vi "TeachAndPlay_old.vi"() -> ()   [LabVIEW 2013]
uses:
  ROS/Code/JointPositions.ctl
  ROS/Code/SubVIs/BaxterSide.ctl
  ROS/Code/SubVIs/BaxterButtons.ctl
panel:
  in  "Functions":i32[](listbox)=[0, 2, 4]
  out "Gripper State":bool=TRUE
  in  "Path":T2(array[cluster])=[{"Position"={"e0"=0.043945312449785154, "e1"=0.417480468272959, "s0"=0.08789062489957031, "s1"=0.8569335927708106, "w0"=0.08789062489957031, "w1"=0.1318359373493555, "w2"=-0.1098632811244629}, "Name"="Zero", "Gripper"=TRUE}, {"Position"={"e0"=1.6918945293167287, "e1"=3.4497070273081354, "s0"=-1.8017578104411913, "s1"=-4.85595702570126, "w0"=0.06591796867467775, "w1"=87.01171865057462, "w2"=0.2416992184738184}, "Name"="Point Down", "Gripper"=TRUE}, {"Position"={"e0"=3.0, "e1"=26.0, "s0"=-51.0, "s1"=-15.0, "w0"=-4.0, "w1"=77.0, "w2"=-4.0}, "Name"="", "Gripper"=FALSE}, {"Position"={"e0"=3.229980465059209, "e1"=26.257324188746633, "s0"=-51.39404291002375, "s1"=-14.63378904577846, "w0"=-3.7573242144566312, "w1"=76.61865225620042, "w2"=-3.6254882771072756}, "Name"="Approach", "Gripper"=TRUE}, {"Position"={"e0"=4.965820306825724, "e1"=34.760742147780064, "s0"=-53.085937439340476, "s1"=-15.754394513247982, "w0"=-3.999023432930449, "w1"=65.06103508190692, "w2"=-3.889160151805987}, "Name"="Grip", "Gripper"=TRUE}, {"Position"={"e0"=4.987792963050616, "e1"=34.89257808512942, "s0"=-53.21777337668983, "s1"=-15.644531232123517, "w0"=-4.08691405783002, "w1"=65.21484367548118, "w2"=-3.823242183131309}, "Name"="Close", "Gripper"=FALSE}, {"Position"={"e0"=7.031249991965626, "e1"=34.9584960538041, "s0"=-53.085937439340476, "s1"=-26.696777313244485, "w0"=-3.889160151805987, "w1"=74.6191405397352, "w2"=-3.8012695269064167}, "Name"="Withdraw", "Gripper"=FALSE}, {"Position"={"e0"=9.03076170843085, "e1"=46.01074213492506, "s0"=-1.2524414048188772, "s1"=-34.69482417910538, "w0"=-12.76611326666259, "w1"=74.59716788351031, "w2"=9.140624989555315}, "Name"="Swing Away", "Gripper"=FALSE}, {"Position"={"e0"=8.898925771081496, "e1"=45.79101557267614, "s0"=-1.2524414048188772, "s1"=-34.541015585531134, "w0"=-12.875976547787051, "w1"=74.75097647708456, "w2"=9.008789052205957}, "Name"="Drop", "Gripper"=TRUE}] {"Position"."w2" scale=-175.25..175.25; "Position"."w1" scale=-90.0..120.0; "Position"."w0" scale=-175.25..175.25; "Position"."e1" scale=-3.0..150.0; "Position"."e0" scale=-173.5..173.5; "Position"."s1" scale=-123.0..60.0; "Position"."s0" scale=-141.0..51.0}
  in  "Tab":enum32{"Teach", "Edit", "Play", "Save", "Load"}(tab)=enum."Play"
  in  "New Path?":bool
  out "Last Activity":string="---------"
  in  "Pause":bool=TRUE
  in  "Tolerance":dbl=1.0
  in  "Settle Time":u32=2500
  in  "save path":path=path "C:/Program Files/Labview/user.lib/ROSforLV_0.1/Devices/Baxter/Baxter Examples/Paths/Pick.csv"
  in  "Save":bool
  in  "load file":path
  in  "Load":bool
  in  "stop":bool
  # "Not yet"
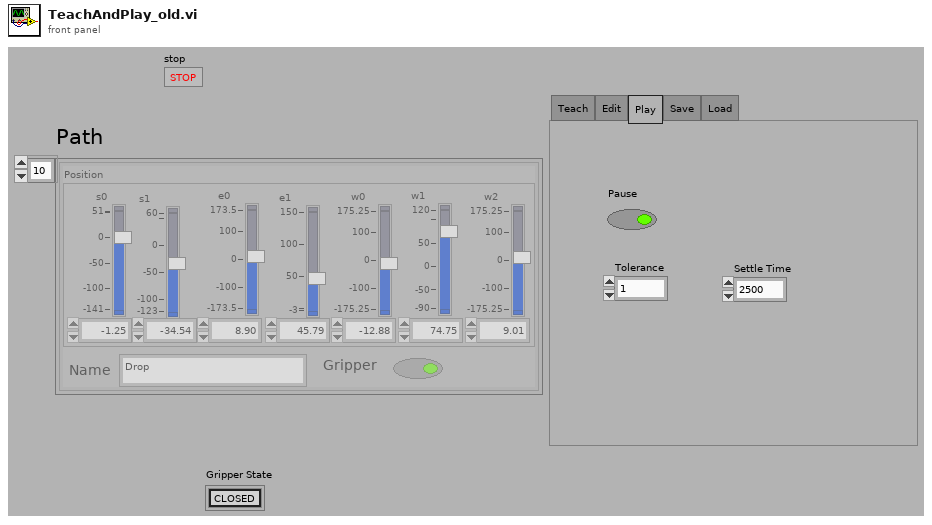
[diagram p1: front panel]
types:
  T1 = typedef "JointPositions.ctl" = cluster{"e0":dbl, "e1":dbl, "s0":dbl, "s1":dbl, "w0":dbl, "w1":dbl, "w2":dbl}
  T2 = cluster{"Position":T1, "Name":string, "Gripper":bool}[]
  T3 = cluster{"Positions":T1, "Name":string, "Gripper":bool}
  T4 = typedef "BaxterSide.ctl" = enum16{"left", "right"}
  T5 = enum16{"open", "replace", "create", "open or create", "replace or create", "replace or create with confirmation"}
  T6 = typedef "BaxterButtons.ctl" = u16
  T7 = cluster{"Cancel":bool, "OK":bool, "Show":bool, "Wheel":u8}
  T8 = cluster{"Positions":T1, "Name":string, "Gripper":bool}[]
  T9 = cluster{"Position":T1, "Name":string, "Gripper":bool}
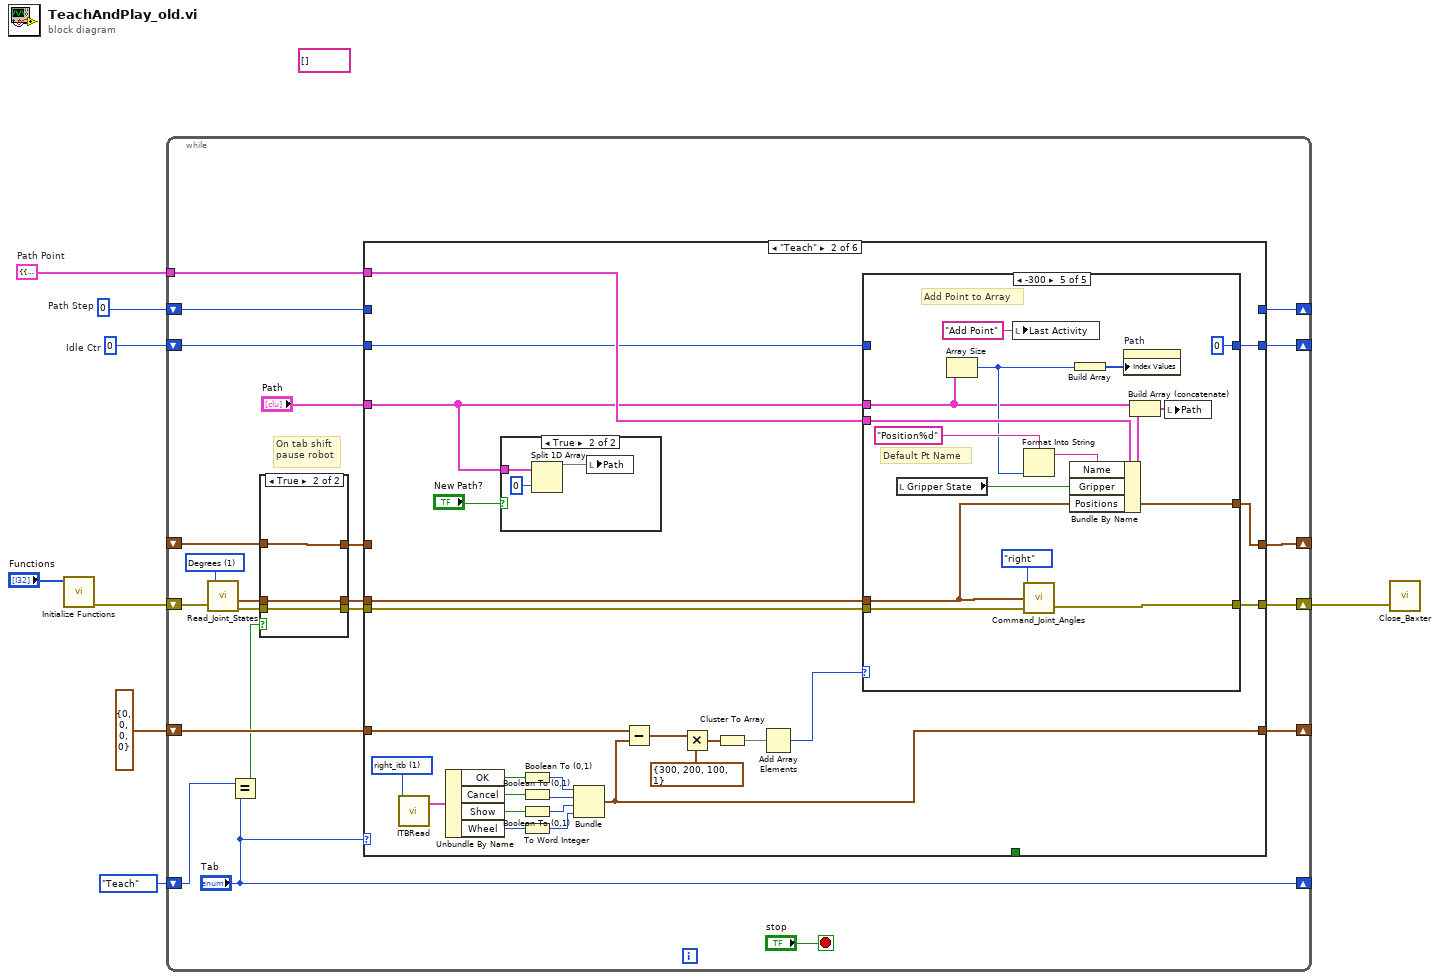
[diagram p0: block diagram]
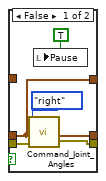
[diagram p2: hidden frame]
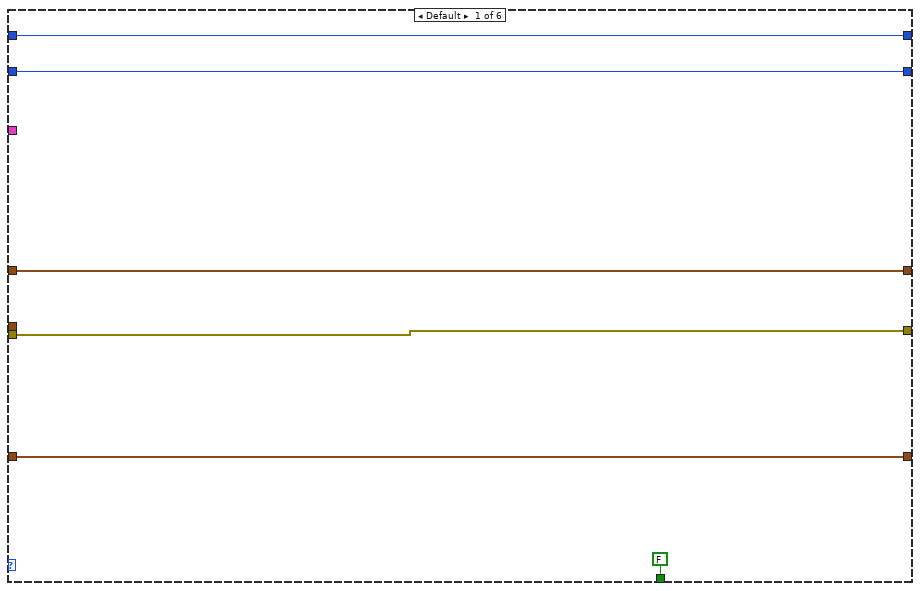
[diagram p3: hidden frame]
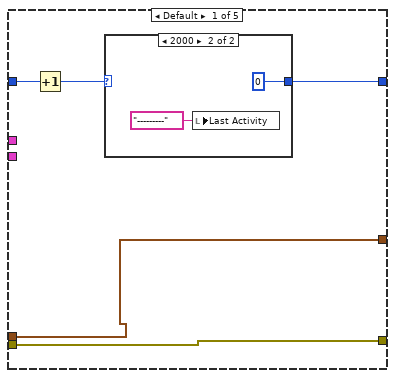
[diagram p5: hidden frame]
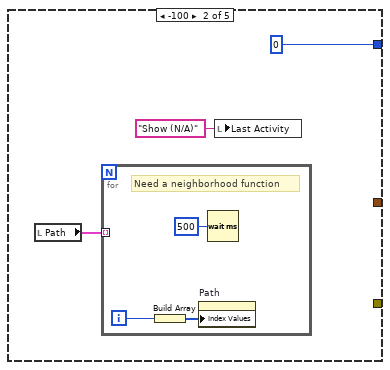
[diagram p7: hidden frame]
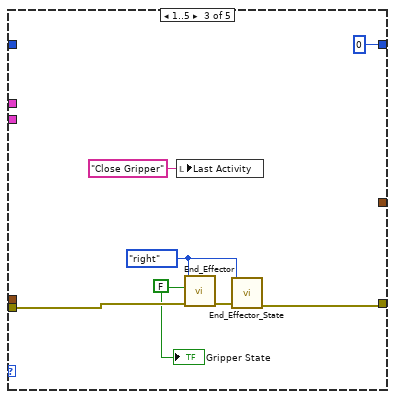
[diagram p8: hidden frame]
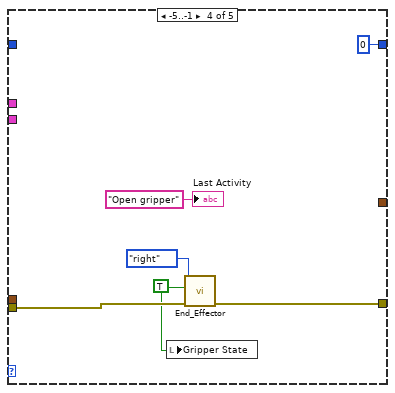
[diagram p9: hidden frame]
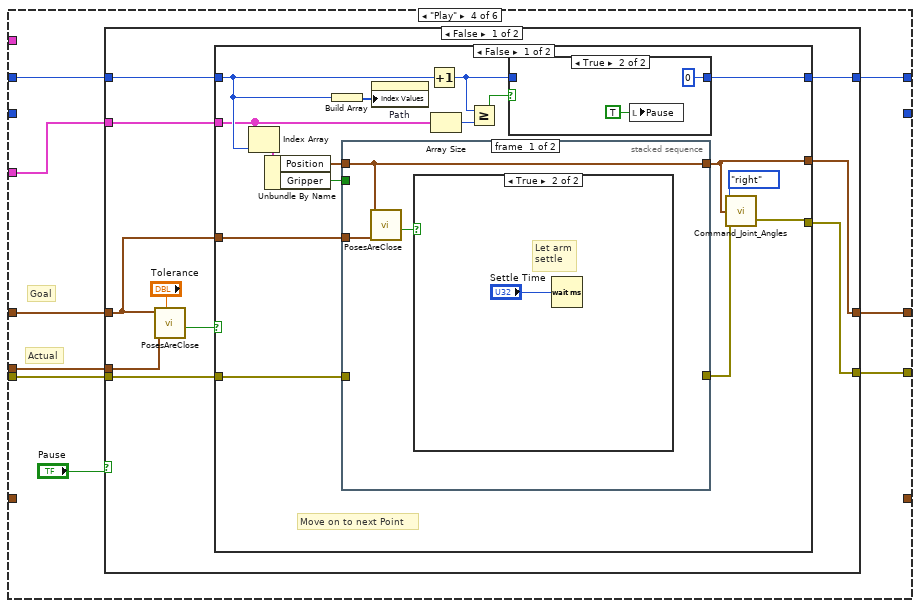
[diagram p11: hidden frame]
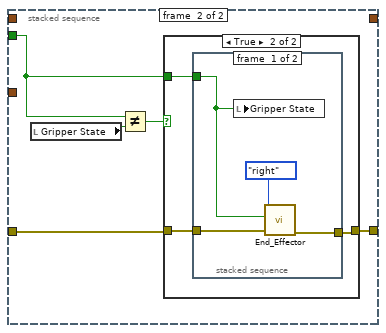
[diagram p13: hidden frame]
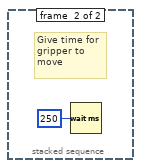
[diagram p15: hidden frame]
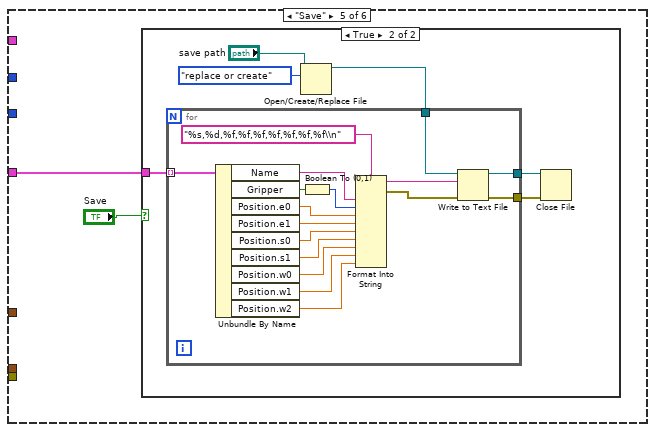
[diagram p19: hidden frame]
diagram:
  w2 = 0  # Path Step
  w4 = 0  # Idle Ctr
  w6 = T3 {"Positions"={"e0"=0.0, "e1"=0.0, "s0"=0.0, "s1"=0.0, "w0"=0.0, "w1"=0.0, "w2"=0.0}, "Name"="", "Gripper"=FALSE}  # Path Point
  (unwired) string[] [] ("Item Names")
  n1 = call "Initialize Functions.vi"("Functions"="Functions") -> ("error out"=w8:errorcluster)  [unwired: 10 in]
  n2 = while {
    shift-right: [w29] -> _
    shift-left: cluster{i16, i16, i16, i16} {0, 0, 0, 0} -> [w30]
    tunnel: w6 -> [w28]
    shift-right: [w27] -> w5
    shift-left: w8 -> [w23]
    shift-right: [w25] -> _
    shift-left: w4 -> [w26]
    shift-right: ["Tab"] -> _
    shift-left: enum32{"Teach", "Edit", "Run", "Save", "Load"}."Teach" ("Tab") -> [w22]
    shift-right: [w15] -> _
    shift-left: _ -> [w12]
    shift-right: [w10] -> _
    shift-left: w2 -> [w14]
    stop <- "stop" stop-if-true
    w24 = u16 1 items=["Radians", "Degrees"] ("Units (Rad)")
    # "On tab shift\npause robot"
    n3 = call "Read_Joint_States.vi"("Units (deg)"=w24, "error in"=w23) -> ("right Positions"=w18:T1, "error out"=w19:errorcluster)  [unwired: 2 in, 2 out]
    n4 = Equal?(x=w22, y="Tab") -> (x = y?=w20:bool)
    n5 = case shown="True" w20 {
      tunnel: w19 -> [w34 w38]
      tunnel: w18 -> [w31 w36]
      tunnel: [w33 w38] -> w17
      tunnel: [w31 w36] -> w16
      tunnel: w12 -> [_ w37]
      tunnel: [w31 w37] -> w11
      frame False {
        n6 = call "Command_Joint_Angles.vi"("Side"=BaxterSide."right", "Arm Angles (degrees)"=w31, "error in"=w34) -> ("error out"=w33:errorcluster)  [unwired: 3 in]
        n7 = local write "Pause"(TRUE ("Pause")) -> ()
      }
      frame True {
      }
    }
    n8 = case shown="\"Teach\"" "Tab" {
      tunnel: w30 -> [w42 w61 _ _ _ _]
      tunnel: [w42 w60 _ _ _ _] -> w29
      tunnel: w28 -> [_ w53 _ _ _ w204]
      tunnel: w17 -> [w43 w52 _ w122 _ _]
      tunnel: [w43 w51 _ w124 _ _] -> w27
      tunnel: w26 -> [w44 w50 _ _ _ _]
      tunnel: [w44 w49 _ _ _ _] -> w25
      tunnel: [FALSE ("Abort") _ _ _ _ _] -> _
      tunnel: w16 -> [_ w48 _ w123 _ _]
      tunnel: [w39 w47 _ w117 _ _] -> w15
      tunnel: w14 -> [w40 _ _ w119 _ _]
      tunnel: w11 -> [w39 _ _ w120 _ _]
      tunnel: [w40 _ _ w118 _ _] -> w10
      tunnel: "Path" -> [_ w45 _ w116 w179 _]
      frame Default {
      }
      frame "Teach" {
        w70 = T6 1 items=["left_itb", "right_itb", "torso_left_itb", "torso_right_itb"] ("Component")
        n9 = call "ITBRead.vi"("Component"=w70) -> ("ITB"=w69:T7)  [unwired: 2 in, 1 out]
        n10 = Unbundle By Name(w69) -> ("OK"=w68:bool, "Cancel"=w67:bool, "Show"=w66:bool, "Wheel"=w64:u8)
        n11 = case shown="True" "New Path?" {
          tunnel: w45 -> [_ w71]
          frame False {
          }
          frame True {
            n12 = Split 1D Array(array=w71, index=0) -> (first subarray=w73:T2)  [unwired: 1 out]
            n13 = local write "Path"(w73) -> ()
          }
        }
        n14 = Boolean To (0,1)(Boolean=w68) -> (0, 1=w65:i16)
        n15 = Boolean To (0,1)(Boolean=w67) -> (0, 1=w62:i16)
        n16 = Boolean To (0,1)(Boolean=w66) -> (0, 1=w63:i16)
        n17 = To Word Integer(number=w64) -> (16bit integer=w59:i16)
        n18 = Bundle(w65, w62, w63, w59) -> (w60:cluster{i16, i16, i16, i16})  [unwired: 1 in]
        n19 = Subtract(x=w61, y=w60) -> (x-y=w58:cluster{i16, i16, i16, i16})
        n20 = Multiply(x=w58, y=cluster{i16, i16, i16, i16} {300, 200, 100, 1}) -> (x*y=w56:cluster{i16, i16, i16, i16})
        n21 = Cluster To Array(cluster=w56) -> (array=w55:i16[])
        n22 = Add Array Elements(numeric array=w55) -> (sum=w54:i16)
        n23 = case shown="-300" w54 {
          tunnel: w53 -> [_ _ _ _ w113]
          tunnel: w52 -> [w78 _ w94 w99 w104]
          tunnel: [w78 _ w90 w98 w112] -> w51
          tunnel: w50 -> [w77 _ _ _ _]
          tunnel: [w75 0 0 0 0] -> w49
          tunnel: w48 -> [w74 _ _ _ w103]
          tunnel: [w74 _ _ _ w103] -> w47
          tunnel: w45 -> [_ _ _ _ w102]
          frame Default {
            n24 = Increment(x=w77) -> (x+1=w76:i32)
            n25 = case shown="2000" w76 {
              selector: w76 -> [w79 _]
              tunnel: [w79 0] -> w75
              frame 0, Default {
              }
              frame 2000 {
                n26 = local write "Last Activity"("---------" ("Last Activity")) -> ()
              }
            }
          }
          frame -100 {
            n27 = local read "Path"() -> (w82:T2)
            n28 = for {
              tunnel: w82 -> [_] mode=indexing
              i -> [w87]
              # "Need a neighborhood function"
              n29 = Build Array(w87) -> (w86:i32[])
              n30 = property on="Path" class="Arr (strict)"("Index Values"=w86) -> ()  [unwired: 2 in, 2 out]
              n31 = Wait (ms)(milliseconds to wait=u32 500) -> ()  [unwired: 1 out]
            }
            n32 = local write "Last Activity"("Show (N/A)" ("Last Activity")) -> ()
          }
          frame 1..5 {
            w89 = BaxterSide."right" ("Side")
            w88 = FALSE ("Calibrate")
            n33 = local write "Last Activity"("Close Gripper" ("Last Activity")) -> ()
            n34 = call "End_Effector.vi"("error in"=w94, "Open"=w88, "Side"=w89) -> ("error out"=w91:errorcluster)  [unwired: 5 in]
            n35 = call "End_Effector_State.vi"("Side"=w89, "error in"=w91) -> ("error out"=w90:errorcluster)  [unwired: 4 in]
            "Gripper State" <- w88
          }
          frame -5..-1 {
            w95 = TRUE ("Calibrate")
            n36 = local write "Gripper State"(w95) -> ()
            n37 = call "End_Effector.vi"("error in"=w99, "Open"=w95, "Side"=BaxterSide."right") -> ("error out"=w98:errorcluster)  [unwired: 5 in]
            "Last Activity" <- "Open gripper" ("Last Activity")
          }
          frame -300 {
            # "Default Pt Name"
            # "Add Point to Array"
            n38 = local read "Gripper State"() -> (w101:bool)
            n39 = Array Size(array=w102) -> (size(s)=w106:i32)
            n40 = local write "Last Activity"("Add Point" ("Last Activity")) -> ()
            n41 = Format Into String(format string="Position%d" ("Name"), w106) -> (resulting string=w105:string)  [unwired: 2 in, 1 out]
            n42 = call "Command_Joint_Angles.vi"("Side"=BaxterSide."right", "Arm Angles (degrees)"=w103, "error in"=w104) -> ("error out"=w112:errorcluster)  [unwired: 3 in]
            n43 = Bundle By Name(cluster=w113, "Name"=w105, "Gripper"=w101, "Positions"=w103) -> (w114:T3)
            n44 = Build Array(w106) -> (w108:i32[])
            n45 = property on="Path" class="Arr (strict)"("Index Values"=w108) -> ()  [unwired: 2 in, 2 out]
            n46 = Build Array (concatenate)(w102, w114) -> (w109:T8)
            n47 = local write "Path"(w109) -> ()
          }
        }
      }
      frame "Edit" {
      }
      frame "Play" {
        # "Actual"
        # "Goal"
        n48 = case shown="False" "Pause" {
          tunnel: [w130 w176] -> w124
          tunnel: w123 -> [w127 _]
          tunnel: w122 -> [w131 w176]
          tunnel: w120 -> [w128 w175]
          tunnel: w119 -> [w134 w177]
          tunnel: [w133 w177] -> w118
          tunnel: [w132 w175] -> w117
          tunnel: w116 -> [w129 _]
          frame False {
            n49 = call "PosesAreClose.vi"("Tolerance"="Tolerance", "Position 2"=w127, "Position"=w128) -> ("Close"=w125:bool)  [unwired: 8 in]
            n50 = case shown="False" w125 {
              tunnel: w134 -> [w140 w173]
              tunnel: [w141 w173] -> w133
              tunnel: [w135 w174] -> w132
              tunnel: w128 -> [w136 w174]
              tunnel: w131 -> [w149 w172]
              tunnel: [w147 w172] -> w130
              tunnel: w129 -> [w138 _]
              frame False {
                # "Move on to next Point"
                n51 = Index Array(array=w138, index=w140) -> (element=w150:T9)
                n52 = Unbundle By Name(w150) -> ("Position"=w137:T1, "Gripper"=w148:bool)
                n53 = Build Array(w140) -> (w139:i32[])
                n54 = stacked-sequence {
                  tunnel: w149 -> [_ w158]
                  tunnel: w148 -> [_ w156]
                  tunnel: [_ w155] -> w146
                  tunnel: w137 -> [w151 _]
                  tunnel: w136 -> [w153 _]
                  tunnel: [w151 _] -> w135
                  frame #0 {
                    n55 = call "PosesAreClose.vi"("Position 2"=w153, "Position"=w151) -> ("Close"=w152:bool)  [unwired: 9 in]
                    n56 = case shown="True" w152 {
                      frame False {
                      }
                      frame True {
                        # "Let arm\nsettle"
                        n57 = Wait (ms)(milliseconds to wait="Settle Time") -> ()  [unwired: 1 out]
                      }
                    }
                  }
                  frame #1 {
                    n58 = local read "Gripper State"() -> (w159:bool)
                    n59 = Not Equal?(x=w156, y=w159) -> (x != y?=w157:bool)
                    n60 = case shown="True" w157 {
                      tunnel: w158 -> [w160 w163]
                      tunnel: w156 -> [_ w162]
                      tunnel: [w160 w161] -> w155
                      frame False {
                      }
                      frame True {
                        n61 = stacked-sequence {
                          tunnel: w163 -> [w166 _]
                          tunnel: w162 -> [w164 _]
                          tunnel: [w165 _] -> w161
                          frame #0 {
                            n62 = local write "Gripper State"(w164) -> ()
                            n63 = call "End_Effector.vi"("error in"=w166, "Open"=w164, "Side"=BaxterSide."right") -> ("error out"=w165:errorcluster)  [unwired: 5 in]
                          }
                          frame #1 {
                            # "Give time for\ngripper to\nmove"
                            n64 = Wait (ms)(milliseconds to wait=u32 250) -> ()  [unwired: 1 out]
                          }
                        }
                      }
                    }
                  }
                }
                n65 = property on="Path" class="Arr (strict)"("Index Values"=w139) -> ()  [unwired: 2 in, 2 out]
                n66 = Increment(x=w140) -> (x+1=w142:i32)
                n67 = Array Size(array=w138) -> (size(s)=w144:i32)
                n68 = Greater Or Equal?(x=w142, y=w144) -> (x >= y?=w143:bool)
                n69 = case shown="True" w143 {
                  tunnel: w142 -> [w169 _]
                  tunnel: [w169 0] -> w141
                  frame False {
                  }
                  frame True {
                    n70 = local write "Pause"(TRUE ("Pause")) -> ()
                  }
                }
                n71 = call "Command_Joint_Angles.vi"("Side"=BaxterSide."right", "Arm Angles (degrees)"=w135, "error in"=w146) -> ("error out"=w147:errorcluster)  [unwired: 3 in]
              }
              frame True {
                # "Not within Tolerance\nLet Robot Run"
              }
            }
          }
          frame True {
            # "Paused\n\nDo Nothing!!!"
          }
        }
      }
      frame "Save" {
        n72 = case shown="True" "Save" {
          tunnel: w179 -> [_ w185]
          frame False {
          }
          frame True {
            n73 = Open/Create/Replace File(file path (use dialog)="save path", operation (0:open)=T5."replace or create") -> (refnum out=w184:refnum<file>)  [unwired: 4 in, 2 out]
            n74 = for {
              tunnel: w185 -> [w202] mode=indexing
              tunnel: [w188] -> w183
              tunnel: w184 -> [w187]
              tunnel: [w186] -> w182
              n75 = Unbundle By Name(w202) -> ("Name"=w198:string, "Gripper"=w200:bool, "Position.e0"=w197:dbl, "Position.e1"=w196:dbl, "Position.s0"=w195:dbl, "Position.s1"=w194:dbl, "Position.w0"=w193:dbl, "Position.w1"=w192:dbl, "Position.w2"=w191:dbl)
              n76 = Boolean To (0,1)(Boolean=w200) -> (0, 1=w199:i16)
              n77 = Format Into String(format string="%s,%d,%f,%f,%f,%f,%f,%f,%f\\n", w198, w199, w197, w196, w195, w194, w193, w192, w191) -> (resulting string=w190:string, error out=w189:errorcluster)  [unwired: 2 in]
              n78 = Write to Text File(file (use dialog)=w187, text=w190, error in=w189) -> (refnum out=w186:refnum<file>, error out=w188:errorcluster)  [unwired: 1 in, 1 out]
            }
            n79 = Close File(refnum=w182, error in=w183) -> ()  [unwired: 2 out]
          }
        }
      }
      frame "Load" {
        n80 = case shown="True" "Load" {
          tunnel: w204 -> [_ w208]
          frame False {
          }
          frame True {
            n81 = Open/Create/Replace File(file path (use dialog)="load file", operation (0:open)=T5."open") -> (refnum out=w213:refnum<file>, error out=w211:errorcluster)  [unwired: 4 in, 1 out]
            n82 = Read from Text File(file (use dialog)=w213, count=-1, error in=w211) -> (refnum out=w212:refnum<file>, text=w206:string[], error out=w210:errorcluster)  [unwired: 1 in, 1 out]
            n83 = Close File(refnum=w212, error in=w210) -> (error out=w205:errorcluster)  [unwired: 1 out]
            n84 = for {
              tunnel: w206 -> [w228] mode=indexing
              tunnel: w208 -> [w231]
              tunnel: [w230] -> w207 mode=indexing
              tunnel: [w229] -> _
              tunnel: w205 -> [w216]
              n85 = Match Pattern(string=w228, regular expression=",") -> (before substring=w225:string, after substring=w226:string)  [unwired: 1 in, 2 out]
              n86 = Scan From String(format string="%d,%f,%f,%f,%f,%f,%f,%f", input string=w226, error in=w216) -> (error out=w229:errorcluster, output 1=w224:i32, output 2=w223:dbl, output 3=w222:dbl, output 4=w221:dbl, output 5=w220:dbl, output 6=w219:dbl, output 7=w218:dbl, output 8=w217:dbl)  [unwired: 9 in, 2 out]
              n87 = Greater Than 0?(x=w224) -> (x > 0?=w232:bool)
              n88 = Bundle By Name(cluster=w231, "Name"=w225, "Gripper"=w232, "Positions.e0"=w223, "Positions.e1"=w222, "Positions.s0"=w221, "Positions.s1"=w220, "Positions.w0"=w219, "Positions.w1"=w218, "Positions.w2"=w217) -> (w230:T3)
            }
            n89 = local write "Path"(w207) -> ()
          }
        }
      }
    }
  }
  n90 = call "Close_Baxter.vi"("error in"=w5) -> ()  [unwired: 3 in, 1 out]
